vi "FindPivotSystemErrors.vi"(10 "Desired Motion":T1, 11 "Actual Pivot System":T1) -> (3 "Commanded Motion":T1)   [LabVIEW 2019]
uses:
  Controls/Robot Pivot Motion Commands.ctl
  Controls/Pivot Motor Commands.ctl
  Controls/Robot Drive Mode.ctl
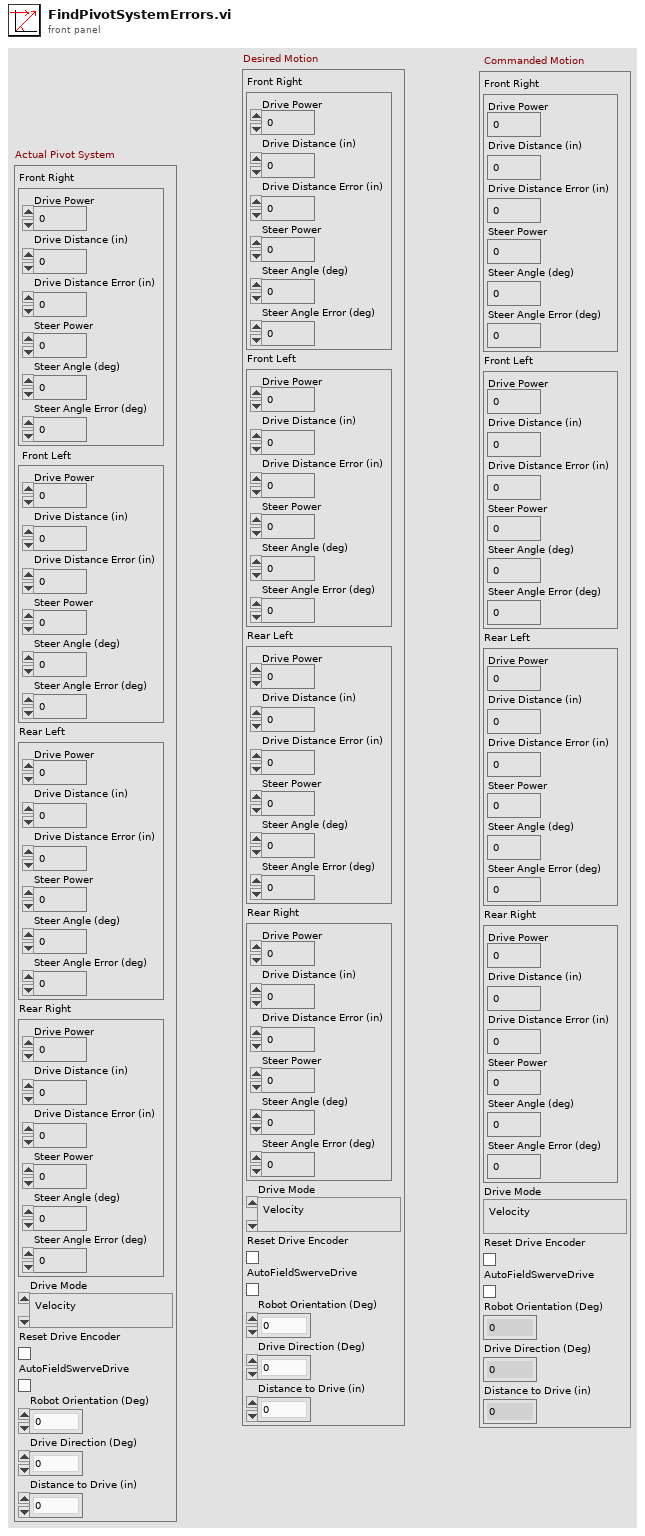
[diagram p1: front panel]
types:
  T1 = typedef "Robot Pivot Motion Commands.ctl" = cluster{"Front Right":T2, "Front Left":T2, "Rear Left":T2, "Rear Right":T2, "Drive Mode":T3, "Reset Drive Encoder":bool, "AutoFieldSwerveDrive":bool, "Robot Orientation (Deg)":dbl, "Drive Direction (Deg)":dbl, "Distance to Drive (in)":dbl}
  T2 = typedef "Pivot Motor Commands.ctl" = cluster{"Drive Power":dbl, "Drive Distance (in)":dbl, "Drive Distance Error (in)":dbl, "Steer Power":dbl, "Steer Angle (deg)":dbl, "Steer Angle Error (deg)":dbl}
  T3 = typedef "Robot Drive Mode.ctl" = enum16{"Velocity", "Distance"}
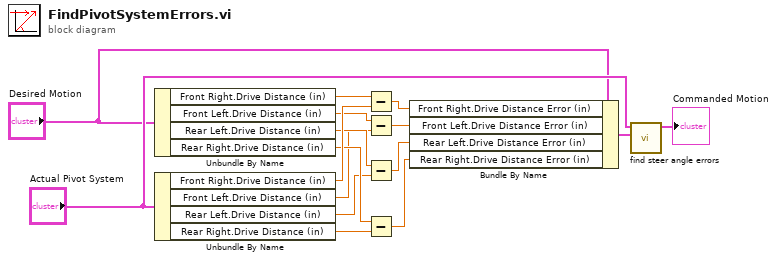
[diagram p0: block diagram]
diagram:
  n1 = Unbundle By Name("Desired Motion") -> ("Front Right.Drive Distance (in)"=w12:dbl, "Front Left.Drive Distance (in)"=w10:dbl, "Rear Left.Drive Distance (in)"=w9:dbl, "Rear Right.Drive Distance (in)"=w8:dbl)
  n2 = Unbundle By Name("Actual Pivot System") -> ("Front Right.Drive Distance (in)"=w11:dbl, "Front Left.Drive Distance (in)"=w7:dbl, "Rear Left.Drive Distance (in)"=w6:dbl, "Rear Right.Drive Distance (in)"=w5:dbl)
  n3 = Subtract(x=w12, y=w11) -> (x-y=w4:dbl)
  n4 = Subtract(x=w10, y=w7) -> (x-y=w3:dbl)
  n5 = Subtract(x=w9, y=w6) -> (x-y=w2:dbl)
  n6 = Subtract(x=w8, y=w5) -> (x-y=w1:dbl)
  n7 = Bundle By Name(cluster="Desired Motion", "Front Right.Drive Distance Error (in)"=w4, "Front Left.Drive Distance Error (in)"=w3, "Rear Left.Drive Distance Error (in)"=w2, "Rear Right.Drive Distance Error (in)"=w1) -> (w13:T1)
  n8 = call "find steer angle errors.vi"("Desired Motion"=w13, "Actual Angles"="Actual Pivot System") -> ("Commanded Motion"=→"Commanded Motion":T1)  [unwired: 9 in]
